vi "Create New.vi"(8 "error in (no error)":errorcluster, 10 "DigNum Refnum":refnum<vi>) -> (0 "error out":errorcluster, 3 "Example Step One out":refnum<class "Example Step One.lvclass">)   [LabVIEW 2015, in "Mediator.lvlib" / "Example Step One.lvclass"]
uses:
  Example Step One.lvclass
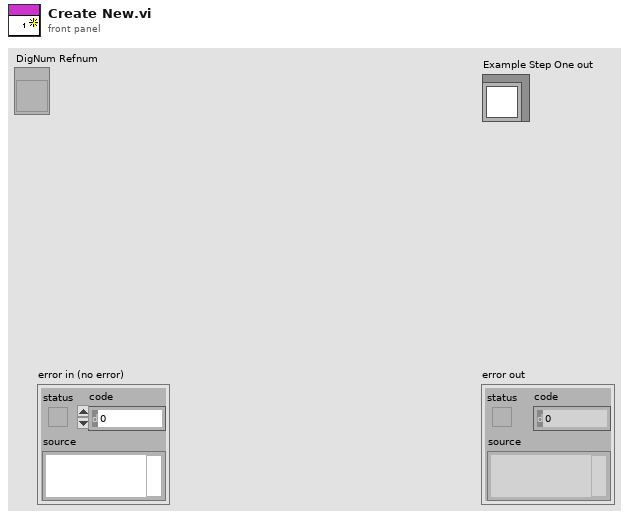
[diagram p1: front panel]
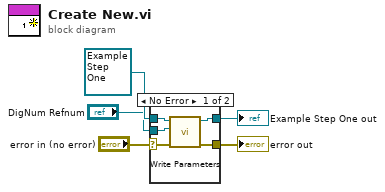
[diagram p0: block diagram]
diagram:
  n1 = case shown="No Error" "error in (no error)" {
    selector: "error in (no error)" -> [w8 w12]
    tunnel: [w7 w12] -> w4
    tunnel: [w9 w11] -> w2
    tunnel: refnum<class "Example Step One.lvclass"> refnum ("Example Step One in") -> [w10 w11]
    tunnel: "DigNum Refnum" -> [w6 _]
    frame No Error {
      n2 = call-dynamic "Write Parameters.vi"("error in (no error)"=w8, "Parameters"=w6, "Step in"=w10) -> ("error out"=w7:errorcluster, "Step out"=w9:refnum<class "Example Step One.lvclass">)  [unwired: 7 in]
    }
    frame Error {
    }
  }
  "error out" <- w4
  "Example Step One out" <- w2
